vi "Increment Build Number.vi"(0 "NI Build Specification in":refnum<class "NI Build Specification_LV.lvclass">, 11 "error in (no error)":errorcluster) -> (4 "NI Build Specification out":refnum<class "NI Build Specification_LV.lvclass">, 15 "error out":errorcluster)   [LabVIEW 2017, in "CL_G3_VIComponentBuilder.lvlib" / "NI Build Specification_LV.lvclass"]
doc: "Increments the build number of the build spec."
uses:
  NI Build Specification_LV.lvclass
  NI Build Specification_LV.lvclass/NI Build Specification_LV.ctl
  Accessors/Read Project Reference.vi
  Accessors/Read Export's Build Spec Name.vi
  Accessors/Read Target Name Containing Build Specs to Build.vi
  <vilib>/AppBuilder/AB_API_Simple/Get Build Specification Version (project reference).vi
  <vilib>/AppBuilder/AB_API_Simple/Set Build Specification Version (project reference).vi
  <vilib>/AppBuilder/AB_API_Simple/NI_App_Builder_API.lvlib
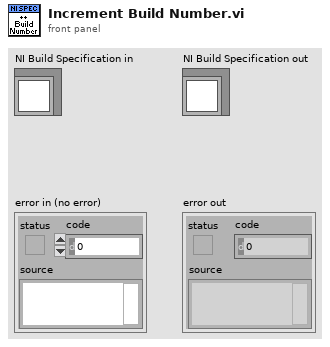
[diagram p1: front panel]
types:
  T1 = typedef "NI_App_Builder_API.lvlib/Build Specification Version.ctl" = cluster{"Major":u16, "Minor":u16, "Fix":u16, "Build":u16}
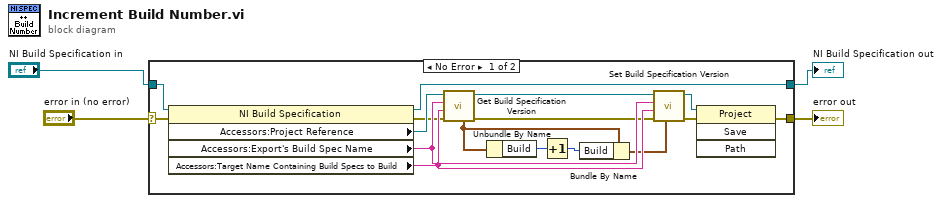
[diagram p0: block diagram]
diagram:
  n1 = case shown="No Error" "error in (no error)" {
    selector: "error in (no error)" -> [w19 w21]
    tunnel: "NI Build Specification in" -> [w20 w22]
    tunnel: [w9 w22] -> w3
    tunnel: [w5 w21] -> w1
    frame No Error {
      n2 = property class="NI Build Specification"(reference=w20, error in=w19) -> (reference out=w9:refnum<class "NI Build Specification_LV.lvclass">, error out=w8:errorcluster, "Accessors:Project Reference"=w18:refnum<vi>, "Accessors:Export's Build Spec Name"=w15:string, "Accessors:Target Name Containing Build Specs to Build"=w16:string)
      n3 = call-poly <vilib>:"Get Build Specification Version.vi"("error in (no error)"=w8, "Name of target (My Computer)"=w16, "Name of build specification"=w15, "Project reference"=w18) -> ("error out"=w12:errorcluster, "dup Project reference"=w17:refnum<vi>, "Build Specification Version"=w6:T1)  [unwired: 5 in]
      n4 = Unbundle By Name(w6) -> ("Build"=w14:u16)
      n5 = Increment(x=w14) -> (x+1=w13:u16)
      n6 = Bundle By Name(cluster=w6, "Build"=w13) -> (w7:T1)
      n7 = call-poly <vilib>:"Set Build Specification Version.vi"("Build Specification Version"=w7, "error in (no error)"=w12, "Name of target (My Computer)"=w16, "Name of build specification"=w15, "Project reference"=w17) -> ("error out"=w10:errorcluster, "dup Project reference"=w11:refnum<vi>)  [unwired: 5 in]
      n8 = invoke class="Project" method="Save"(reference=w11, error in=w10) -> (error out=w5:errorcluster)  [unwired: 2 in, 3 out]
    }
    frame Error {
    }
  }
  "error out" <- w1
  "NI Build Specification out" <- w3
